vi "Read #Pasajeros.vi"(8 "error in (no error)":errorcluster, 11 "Vehiculo de Motor in":refnum<class "Vehiculo de Motor.lvclass">) -> (0 "error out":errorcluster, 2 "#Pasajeros":u16, 3 "Vehiculo de Motor out":refnum<class "Vehiculo de Motor.lvclass">)   [LabVIEW 2020, in "Vehiculo de Motor.lvclass"]
uses:
  Vehiculo de Motor.lvclass
  Vehiculo de Motor.lvclass/Vehiculo de Motor.ctl
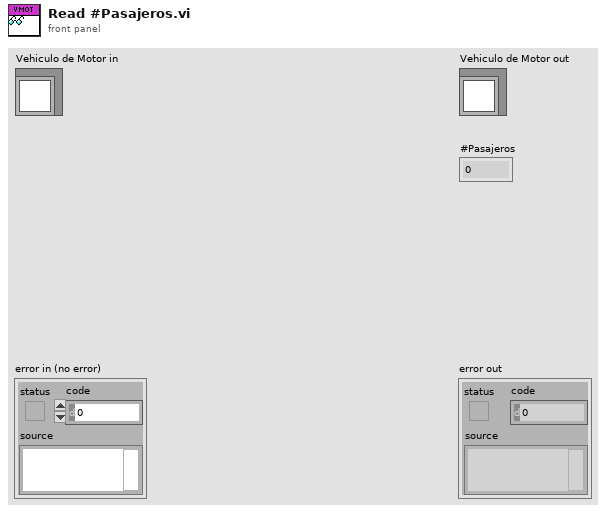
[diagram p1: front panel]
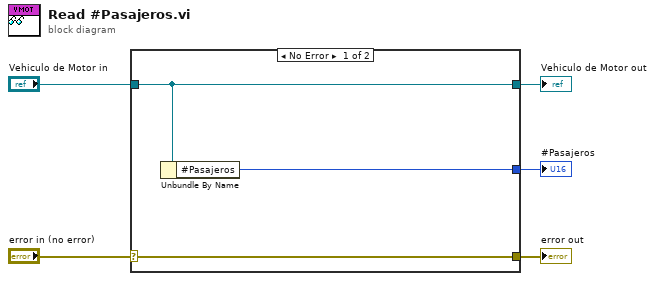
[diagram p0: block diagram]
diagram:
  n1 = case shown="No Error" "error in (no error)" {
    selector: "error in (no error)" -> [w8 w9]
    tunnel: [w8 w9] -> w4
    tunnel: [w7 w10] -> w2
    tunnel: "Vehiculo de Motor in" -> [w7 w10]
    tunnel: [w6 _] -> w1
    frame No Error {
      n2 = Unbundle By Name(w7) -> ("#Pasajeros"=w6:u16)
    }
    frame Error {
    }
  }
  "error out" <- w4
  "Vehiculo de Motor out" <- w2
  "#Pasajeros" <- w1
